vi "Main_10a refactored.vi"() -> ()   [LabVIEW 2020]
panel:
  in  "Puzzle Description":string="--- Day 10: Cathode-Ray Tube ---\nYou avoid the ropes, plunge into the river, and swim to shore.\n\nThe Elves yell something about meeting back up with them upriver, but the river is too loud to tell exactly what they're saying. They finish crossing the bridge and disappear from view.\n\nSituations like this must be why the Elves prioritized getting the communication system on your handheld device working. You pull it out of your pack, but the amount of water slowly draining from a big crack in its screen tells you it probably won't be of much immediate use.\n\nUnless, that is, you can design a replacement for the device's video system! It seems to be some kind of cathode-ray tube screen and simple CPU that are both driven by a precise clock circuit. The clock circuit ticks at a constant rate; each tick is called a cycle.\n\nStart by figuring out the signal being sent by the CPU. The CPU has a single register, X, which starts with the value 1. It supports only two instructions:\n\naddx V takes two cycles to complete. After two cycles, the X register is increased by the value V. (V can be negative.)\nnoop takes one cycle to complete. It has no other effect.\nThe CPU uses these instructions in a program (your puzzle input) to, somehow, tell the screen what to draw.\n\nConsider the following small program:\n\nnoop\naddx 3\naddx -5\nExecution of this program proceeds as follows:\n\nAt the start of the first cycle, the noop instruction begins execution. During the first cycle, X is 1. After the first cycle, the noop instruction finishes execution, doing nothing.\nAt the start of the second cycle, the addx 3 instruction begins execution. During the second cycle, X is still 1.\nDuring the third cycle, X is still 1. After the third cycle, the addx 3 instruction finishes execution, setting X to 4.\nAt the start of the fourth cycle, the addx -5 instruction begins execution. During the fourth cycle, X is still 4.\nDuring the fifth cycle, X is still 4. After the fifth cycle, the addx -5 instruction finishes execution, setting X to -1.\nMaybe you can learn something by looking at the value of the X register throughout execution. For now, consider the signal strength (the cycle number multiplied by the value of the X register) during the 20th cycle and every 40 cycles after that (that is, during the 20th, 60th, 100th, 140th, 180th, and 220th cycles).\n\nFor example, consider this larger program:\n\naddx 15\naddx -11\naddx 6\naddx -3\naddx 5\naddx -1\naddx -8\naddx 13\naddx 4\nnoop\naddx -1\naddx 5\naddx -1\naddx 5\naddx -1\naddx 5\naddx -1\naddx 5\naddx -1\naddx -35\naddx 1\naddx 24\naddx -19\naddx 1\naddx 16\naddx -11\nnoop\nnoop\naddx 21\naddx -15\nnoop\nnoop\naddx -3\naddx 9\naddx 1\naddx -3\naddx 8\naddx 1\naddx 5\nnoop\nnoop\nnoop\nnoop\nnoop\naddx -36\nnoop\naddx 1\naddx 7\nnoop\nnoop\nnoop\naddx 2\naddx 6\nnoop\nnoop\nnoop\nnoop\nnoop\naddx 1\nnoop\nnoop\naddx 7\naddx 1\nnoop\naddx -13\naddx 13\naddx 7\nnoop\naddx 1\naddx -33\nnoop\nnoop\nnoop\naddx 2\nnoop\nnoop\nnoop\naddx 8\nnoop\naddx -1\naddx 2\naddx 1\nnoop\naddx 17\naddx -9\naddx 1\naddx 1\naddx -3\naddx 11\nnoop\nnoop\naddx 1\nnoop\naddx 1\nnoop\nnoop\naddx -13\naddx -19\naddx 1\naddx 3\naddx 26\naddx -30\naddx 12\naddx -1\naddx 3\naddx 1\nnoop\nnoop\nnoop\naddx -9\naddx 18\naddx 1\naddx 2\nnoop\nnoop\naddx 9\nnoop\nnoop\nnoop\naddx -1\naddx 2\naddx -37\naddx 1\naddx 3\nnoop\naddx 15\naddx -21\naddx 22\naddx -6\naddx 1\nnoop\naddx 2\naddx 1\nnoop\naddx -10\nnoop\nnoop\naddx 20\naddx 1\naddx 2\naddx 2\naddx -6\naddx -11\nnoop\nnoop\nnoop\nThe interesting signal strengths can be determined as follows:\n\nDuring the 20th cycle, register X has the value 21, so the signal strength is 20 * 21 = 420. (The 20th cycle occurs in the middle of the second addx -1, so the value of register X is the starting value, 1, plus all of the other addx values up to that point: 1 + 15 - 11 + 6 - 3 + 5 - 1 - 8 + 13 + 4 = 21.)\nDuring the 60th cycle, register X has the value 19, so the signal strength is 60 * 19 = 1140.\nDuring the 100th cycle, register X has the value 18, so the signal strength is 100 * 18 = 1800.\nDuring the 140th cycle, register X has the value 21, so the signal strength is 140 * 21 = 2940.\nDuring the 180th cycle, register X has the value 16, so the signal strength is 180 * 16 = 2880.\nDuring the 220th cycle, register X has the value 18, so the signal strength is 220 * 18 = 3960.\nThe sum of these signal strengths is 13140.\n\nFind the signal strength during the 20th, 60th, 100th, 140th, 180th, and 220th cycles. What is the sum of these six signal strengths?"
  out "Final X":i32
  out "Values of that cycle":i32[](array[numeric])
  in  "Example 2":string="addx 15\naddx -11\naddx 6\naddx -3\naddx 5\naddx -1\naddx -8\naddx 13\naddx 4\nnoop\naddx -1\naddx 5\naddx -1\naddx 5\naddx -1\naddx 5\naddx -1\naddx 5\naddx -1\naddx -35\naddx 1\naddx 24\naddx -19\naddx 1\naddx 16\naddx -11\nnoop\nnoop\naddx 21\naddx -15\nnoop\nnoop\naddx -3\naddx 9\naddx 1\naddx -3\naddx 8\naddx 1\naddx 5\nnoop\nnoop\nnoop\nnoop\nnoop\naddx -36\nnoop\naddx 1\naddx 7\nnoop\nnoop\nnoop\naddx 2\naddx 6\nnoop\nnoop\nnoop\nnoop\nnoop\naddx 1\nnoop\nnoop\naddx 7\naddx 1\nnoop\naddx -13\naddx 13\naddx 7\nnoop\naddx 1\naddx -33\nnoop\nnoop\nnoop\naddx 2\nnoop\nnoop\nnoop\naddx 8\nnoop\naddx -1\naddx 2\naddx 1\nnoop\naddx 17\naddx -9\naddx 1\naddx 1\naddx -3\naddx 11\nnoop\nnoop\naddx 1\nnoop\naddx 1\nnoop\nnoop\naddx -13\naddx -19\naddx 1\naddx 3\naddx 26\naddx -30\naddx 12\naddx -1\naddx 3\naddx 1\nnoop\nnoop\nnoop\naddx -9\naddx 18\naddx 1\naddx 2\nnoop\nnoop\naddx 9\nnoop\nnoop\nnoop\naddx -1\naddx 2\naddx -37\naddx 1\naddx 3\nnoop\naddx 15\naddx -21\naddx 22\naddx -6\naddx 1\nnoop\naddx 2\naddx 1\nnoop\naddx -10\nnoop\nnoop\naddx 20\naddx 1\naddx 2\naddx 2\naddx -6\naddx -11\nnoop\nnoop\nnoop"
  out "sum":i32
  in  "Puzzle":string="addx 1\naddx 5\nnoop\naddx -1\nnoop\naddx 3\naddx 29\naddx -1\naddx -21\naddx 5\nnoop\naddx -20\naddx 21\naddx 2\naddx 8\naddx -1\nnoop\nnoop\nnoop\nnoop\naddx 6\naddx -1\naddx -37\naddx 40\naddx -10\naddx -25\naddx 5\naddx 2\naddx 5\nnoop\nnoop\nnoop\naddx 21\naddx -20\naddx 2\nnoop\naddx 3\naddx 2\naddx -5\naddx 12\naddx 3\nnoop\naddx 2\naddx 3\naddx -2\naddx -37\naddx 1\naddx 5\naddx 3\naddx -2\naddx 2\naddx 29\naddx -22\naddx 13\nnoop\naddx -8\naddx -6\naddx 7\naddx 2\nnoop\naddx 7\naddx -2\naddx 5\naddx 2\naddx -26\naddx -11\nnoop\nnoop\naddx 6\naddx 1\naddx 1\nnoop\naddx 4\naddx 5\nnoop\nnoop\naddx -2\naddx 3\nnoop\naddx 2\naddx 5\naddx 2\naddx -22\naddx 27\naddx -1\naddx 1\naddx 5\naddx 2\nnoop\naddx -39\naddx 22\nnoop\naddx -15\naddx 3\naddx -2\naddx 2\naddx -2\naddx 9\naddx 3\nnoop\naddx 2\naddx 3\naddx -2\naddx 2\nnoop\nnoop\nnoop\naddx 5\naddx -17\naddx 24\naddx -7\naddx 8\naddx -36\naddx 2\naddx 3\naddx 33\naddx -32\naddx 4\naddx 1\nnoop\naddx 5\nnoop\nnoop\naddx 20\naddx -15\naddx 4\nnoop\naddx 1\nnoop\naddx 4\naddx 6\naddx -30\naddx 30\nnoop\nnoop\nnoop\nnoop\nnoop"
  in  "Example":string="noop\naddx 3\naddx -5"
  # "17840"
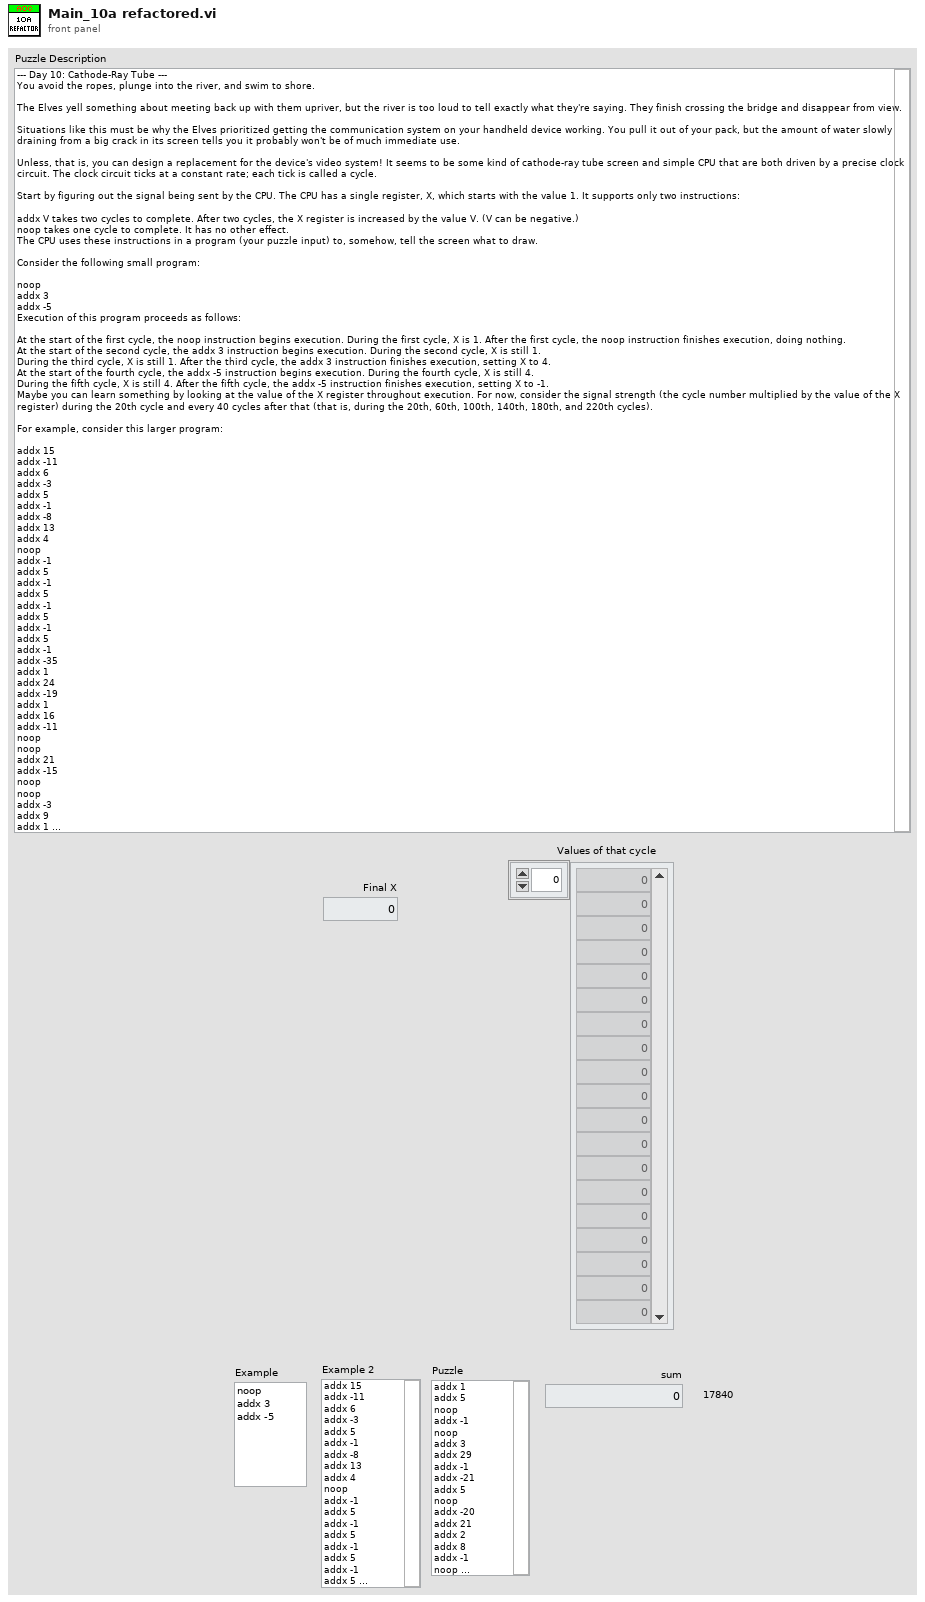
[diagram p1: front panel]
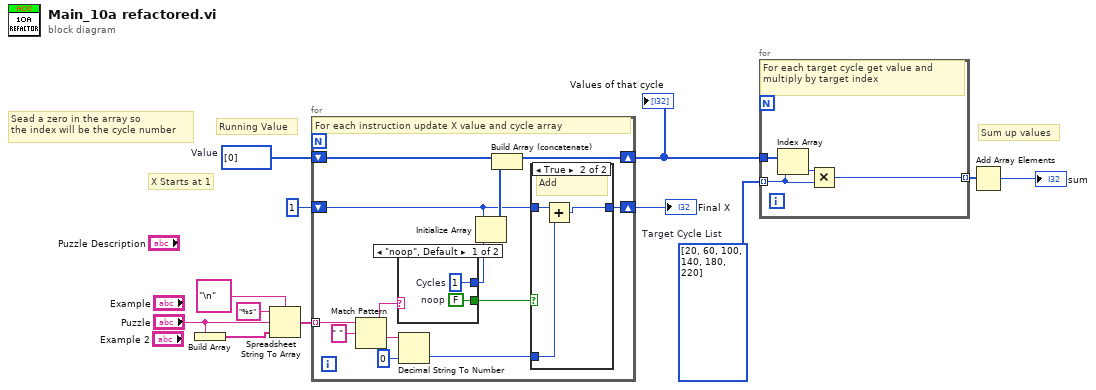
[diagram p0: block diagram]
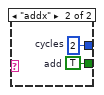
[diagram p2: hidden frame]
diagram:
  w5 = i32[] [20, 60, 100, 140, 180, 220]  # Target Cycle List
  w9 = i32[] [0]  # Value
  # "Sum up values"
  # "Sead a zero in the array so\nthe index will be the cycle number"
  # "X Starts at 1"
  # "Running Value"
  n1 = Build Array("Puzzle") -> (w7:string[])
  n2 = Spreadsheet String To Array(delimiter (Tab)="\n", format string="%s", spreadsheet string="Puzzle", array type (2D Dbl)=w7) -> (array=w8:string[])
  n3 = for {
    shift-right: [w21] -> w6
    shift-left: 1 -> [w23]
    shift-right: [w22] -> w4
    shift-left: w9 -> [w25]
    tunnel: w8 -> [w20] mode=indexing
    # "For each instruction update X value and cycle array"
    n4 = Match Pattern(string=w20, regular expression=" ") -> (before substring=w15:string, after substring=w19:string)  [unwired: 1 in, 2 out]
    n5 = case shown="\"noop\", Default" w15 {
      tunnel: [w27 w29] -> w14
      tunnel: [w26 w28] -> w13
      frame "noop", Default {
        w26 = FALSE  # noop
        w27 = 1  # Cycles
      }
      frame "addx" {
        w28 = TRUE  # add
        w29 = 2  # cycles
      }
    }
    n6 = Decimal String To Number(string=w19, default (0L)=0 ("default (0 I32)")) -> (number=w16:i32)  [unwired: 1 in, 1 out]
    n7 = Initialize Array(w23, w14) -> (w24:i32[])
    n8 = Build Array (concatenate)(w25, w24) -> (w22:i32[])
    n9 = case shown="True" w13 {
      tunnel: w23 -> [w30 w33]
      tunnel: w16 -> [_ w32]
      tunnel: [w30 w31] -> w21
      frame False {
        # "noop"
      }
      frame True {
        # "Add"
        n10 = Add(x=w33, y=w32) -> (x+y=w31:i32)
      }
    }
  }
  "Values of that cycle" <- w4
  "Final X" <- w6
  n11 = for {
    tunnel: w5 -> [w35] mode=indexing
    tunnel: w4 -> [w37]
    tunnel: [w34] -> w3 mode=indexing
    # "For each target cycle get value and multiply by target index"
    n12 = Index Array(array=w37, index=w35) -> (element=w36:i32)
    n13 = Multiply(x=w36, y=w35) -> (x*y=w34:i32)
  }
  n14 = Add Array Elements(numeric array=w3) -> (sum=→"sum":i32)
